vi "AttackPsSkill.vi"(9 "Game in":refnum<class "Game.lvclass">, 10 "Robot":refnum<class "Robot.lvclass">, 11 "AttackPsSkill in":refnum<class "AttackPsSkill.lvclass">) -> (2 "Robot out":refnum<class "Robot.lvclass">, 3 "AttackPsSkill out":refnum<class "AttackPsSkill.lvclass">)   [LabVIEW 2020, in "AttackPsSkill.lvclass"]
uses:
  AttackPsSkill.lvclass
  Robot_class/Robot.lvclass
  C:/Users/User/Documents/GitHub/SSL_AI/Object_class/Object.lvclass
  Game_class/Game.lvclass
  Game_class/Game.lvclass/Game.ctl
  Object_class/Object.lvclass/Object.ctl
  Team_class/Team.lvclass/Team.ctl
  Robot_class/Robot.lvclass/Robot.ctl
  Game_class/Read BallRef.vi
  Game_class/Read FieldRef.vi
  Game_class/Read EnemyRef.vi
  Team_class/Read RobotRef.vi
  Object_class/Read x.vi
  Object_class/Read y.vi
  Robot_class/Write dest_x.vi
  Robot_class/Write dest_y.vi
  Robot_class/Write dest_orientation.vi
  Robot_class/Write kick_x.vi
  Enemy_class/Enemy.lvclass
  C:/Users/User/Documents/GitHub/SSL_AI/Team_class/Team.lvclass
  Ball_class/Ball.lvclass
  Field_class/Field.lvclass
panel:
  out "error out 2":errorcluster
  in  "error in (no error) 2":errorcluster
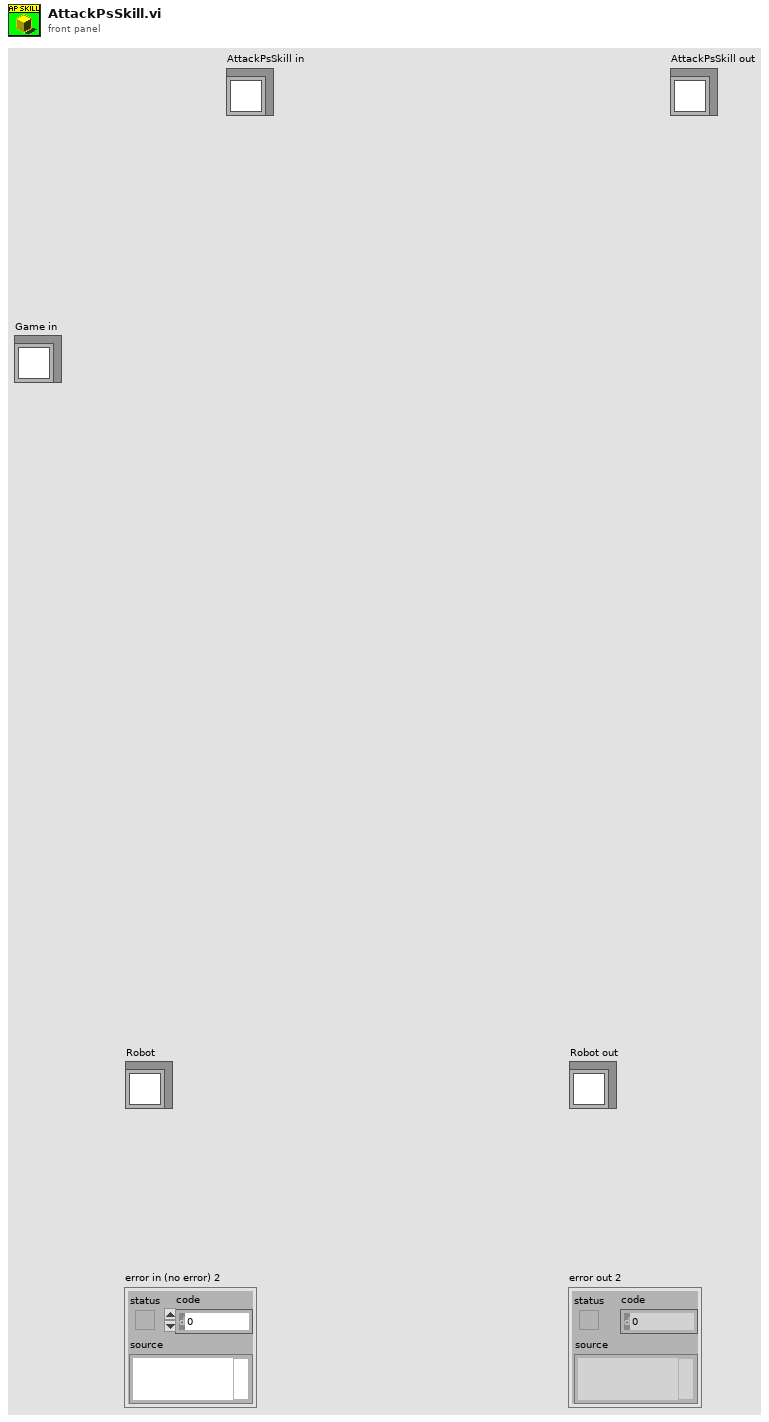
[diagram p1: front panel]
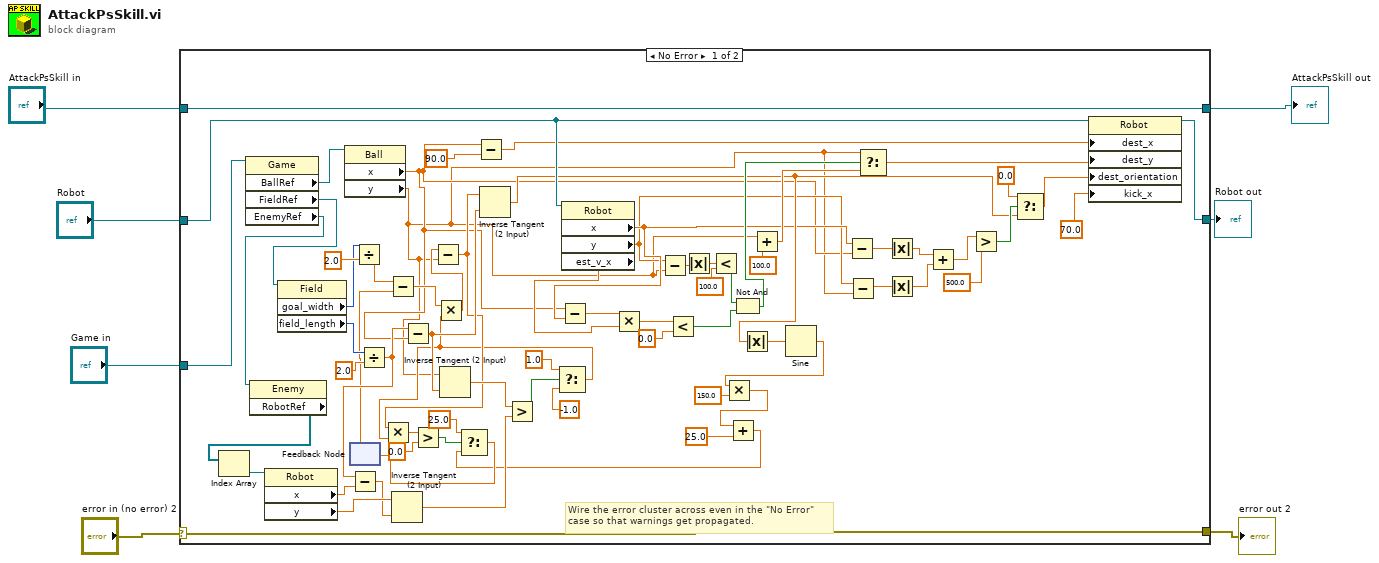
[diagram p0: block diagram]
diagram:
  n1 = case shown="No Error" "error in (no error) 2" {
    selector: "error in (no error) 2" -> [w77 w81]
    tunnel: [w77 w81] -> w6
    tunnel: [w78 w80] -> w3
    tunnel: "AttackPsSkill in" -> [w78 w80]
    tunnel: "Robot" -> [w65 w79]
    tunnel: [w76 w79] -> w4
    tunnel: "Game in" -> [w74 _]
    frame No Error {
      # "Wire the error cluster across even in the \"No Error\"\ncase so that warnings get propagated."
      n2 = property class="Game"(reference=w74) -> ("BallRef"=w73:refnum<class "Ball.lvclass">, "FieldRef"=w72:refnum<class "Field.lvclass">, "EnemyRef"=w51:refnum<class "Enemy.lvclass">)  [unwired: 1 in, 2 out]
      n3 = property class="Enemy"(reference=w51) -> ("RobotRef"=w50:refnum<class "Robot.lvclass">[])  [unwired: 1 in, 2 out]
      n4 = Index Array(array=w50) -> (element=w49:refnum<class "Robot.lvclass">)  [unwired: 1 in]
      n5 = property class="Robot"(reference=w49) -> ("x"=w41:dbl, "y"=w44:dbl)  [unwired: 1 in, 2 out]
      n6 = property class="Field"(reference=w72) -> ("goal_width"=w67:i32, "field_length"=w69:i32)  [unwired: 1 in, 2 out]
      n7 = property class="Ball"(reference=w73) -> ("x"=w9:dbl, "y"=w8:dbl)  [unwired: 1 in, 2 out]
      n8 = feedback #1() -> (w28:dbl)  [unwired: 1 in]
      n9 = Divide(x=w67, y=2.0) -> (x/y=w66:dbl)
      n10 = Divide(x=w69, y=2.0) -> (x/y=w40:dbl)
      n11 = Subtract(x=w40, y=w41) -> (x-y=w43:dbl)
      n12 = Subtract(x=w66, y=w28) -> (x-y=w39:dbl)
      n13 = Inverse Tangent (2 Input)(1:w43, 2:w44) -> (0:w37:dbl)
      n14 = Subtract(x=w40, y=w9) -> (x-y=w45:dbl)
      n15 = Inverse Tangent (2 Input)(1:w45, 2:w8) -> (0:w38:dbl)
      n16 = Subtract(x=w9, y=90.0) -> (x-y=w36:dbl)
      n17 = Greater?(x=w38, y=w37) -> (0:w42:bool)
      n18 = Select(t=1.0, s=w42, f=-1.0) -> (s? t:f=w34:dbl)
      n19 = Multiply(x=w39, y=w34) -> (x*y=w48:dbl)
      n20 = Subtract(x=w48, y=w8) -> (x-y=w35:dbl)
      n21 = Multiply(x=w35, y=w34) -> (x*y=w33:dbl)
      n22 = Greater?(x=w33, y=0.0) -> (0:w31:bool)
      n23 = Inverse Tangent (2 Input)(1:w45, 2:w35) -> (0:w13:dbl)
      n24 = property class="Robot"(reference=w65) -> ("x"=w11:dbl, "y"=w10:dbl, "est_v_x"=w57:dbl)  [unwired: 1 in, 2 out]
      n25 = Subtract(x=w9, y=w11) -> (x-y=w58:dbl)
      n26 = Multiply(x=w58, y=w57) -> (x*y=w59:dbl)
      n27 = Subtract(x=w10, y=w8) -> (x-y=w64:dbl)
      n28 = Less?(x=w59, y=0.0) -> (x < y?=w54:bool)
      n29 = Absolute Value(x=w64) -> (abs(x)=w56:dbl)
      n30 = Less?(x=w56, y=100.0) -> (x < y?=w53:bool)
      n31 = Not And(1:w54, 2:w53) -> (0:w52:bool)
      n32 = Absolute Value(x=w13) -> (abs(x)=w22:dbl)
      n33 = Add(x=w8, y=100.0) -> (x+y=w62:dbl)
      n34 = Sine(x=w22) -> (sin(x)=w23:dbl)
      n35 = Multiply(x=w23, y=150.0) -> (x*y=w26:dbl)
      n36 = Add(x=w26, y=25.0) -> (x+y=w24:dbl)
      n37 = Select(t=25.0, s=w31, f=w24) -> (s? t:f=w29:dbl)
      n38 = feedback-in #1(w29) -> ()
      n39 = Subtract(x=w11, y=w9) -> (x-y=w17:dbl)
      n40 = Subtract(x=w10, y=w8) -> (x-y=w18:dbl)
      n41 = Select(t=w8, s=w52, f=w62) -> (s? t:f=w61:dbl)
      n42 = Absolute Value(x=w17) -> (abs(x)=w21:dbl)
      n43 = Absolute Value(x=w18) -> (abs(x)=w20:dbl)
      n44 = Add(x=w21, y=w20) -> (x+y=w15:dbl)
      n45 = Greater?(x=w15, y=500.0) -> (0:w14:bool)
      n46 = Select(t=0.0, s=w14, f=w13) -> (s? t:f=w12:dbl)
      n47 = property class="Robot"(reference=w65, "dest_x"=w36, "dest_y"=w61, "dest_orientation"=w12, "kick_x"=70.0) -> (reference out=w76:refnum<class "Robot.lvclass">)  [unwired: 1 in, 1 out]
    }
    frame Error {
    }
  }
  "AttackPsSkill out" <- w3
  "error out 2" <- w6
  "Robot out" <- w4
